vi "Advance past Item Name.vi"(7 "JSON":string, 9 "Offset":i32) -> (1 "Offset past colon":i32, 3 "State":T1, 4 "Offset past Name":i32, 6 "Name start out":i32)   [LabVIEW 2019, in "JSONtext.lvlib"]
uses:
  JSONtext.lvlib
  Parsing State.ctl
  Advance past Line Ending.vi
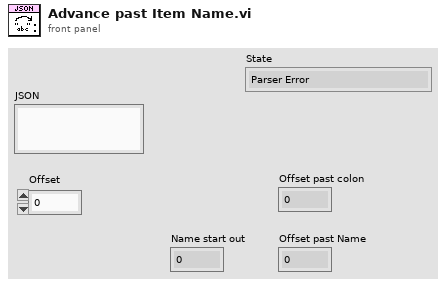
[diagram p1: front panel]
types:
  T1 = typedef "JSONtext.lvlib/Parsing State.ctl" = enum16{"Parser Error", "Object", "Array", "String", "Number/Other", "Leading Whitespace", "Object end", "Array end", "Value end"}
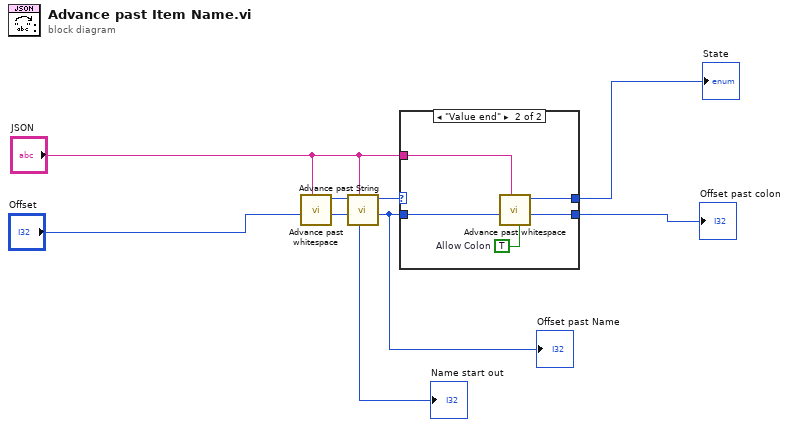
[diagram p0: block diagram]
diagram:
  n1 = call "Advance past whitespace.vi"("JSON"="JSON", "Offset"="Offset") -> ("Offset of first non-whitespace"=w2:i32, "Parser State"=w9:T1)  [unwired: 7 in, 1 out]
  n2 = call "Advance past String.vi"("JSON"="JSON", "Offset"=w2, "State in"=w9) -> ("Offset past match"=w8:i32, "State"=w7:T1, "Value start out"=→"Name start out":i32)  [unwired: 6 in]
  "Offset past Name" <- w8
  n3 = case shown="\"Value end\"" w7 {
    selector: w7 -> [w11 _]
    tunnel: w8 -> [w10 w16]
    tunnel: [w11 w15] -> w6
    tunnel: [w10 w14] -> w5
    tunnel: "JSON" -> [_ w12]
    frame "Parser Error", Default {
    }
    frame "Value end" {
      w13 = TRUE  # Allow Colon
      n4 = call "Advance past whitespace.vi"("Past Colon"=w13, "JSON"=w12, "Offset"=w16) -> ("Offset of first non-whitespace"=w14:i32, "Parser State"=w15:T1)  [unwired: 6 in, 1 out]
    }
  }
  "State" <- w6
  "Offset past colon" <- w5
